vi "New Buffer.vi"(7 "byte order (host order)":T1(ring)=enum."native, host order", 8 "error in (no error)":errorcluster, 9 "buffer offset (0)":u64 format="%d bytes", 10 "buffer size":u64 format="%d bytes", 11 "Buffer type":refnum<class "Buffer.lvclass">) -> (0 "error out":errorcluster, 3 "Buffer out":refnum<class "Buffer.lvclass">)   [LabVIEW 2021, in "DSF Core.lvlib" / "Buffer.lvclass"]
doc: "Allocates a new <b>Buffer</b> of the specified <b>Buffer type</b> that is <b>size</b> bytes in length, and with a set offset at <b>buffer offset</b>.\n\n<b>buffer offset</b> is used with the Align to Base Buffer method to change the location of <b>Buffer</b> to be aligned and offset relative to a provided base Buffer."
uses:
  Buffer.lvclass
  C:/Program Files/National Instruments/LabVIEW 2021/vi.lib/NI/Memory Manager/Classes/Pointer/Pointer.lvclass
  Buffer.lvclass/Buffer.ctl
  <vilib>/NI/Memory Manager/Classes/Pointer/Pointer.lvclass/Pointer.ctl
  <vilib>/NI/Memory Manager/Classes/Pointer/Set Address.vi
  <vilib>/NI/Memory Manager/Classes/Pointer/Set Size.vi
  <vilib>/NI/Memory Manager/Classes/Pointer/Set Internal.vi
  <vilib>/NI/Memory Manager/Classes/Pointer/Pointer.lvclass
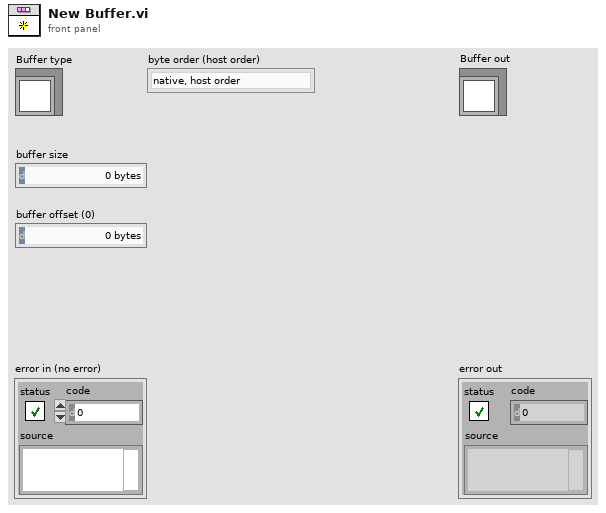
[diagram p1: front panel]
types:
  T1 = enum16{"big-endian, network order", "native, host order", "little-endian"}
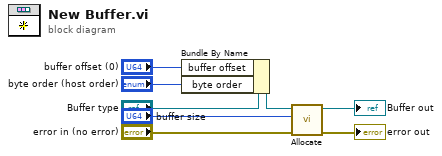
[diagram p0: block diagram]
diagram:
  n1 = Bundle By Name(cluster="Buffer type", "buffer offset"="buffer offset (0)", "byte order"="byte order (host order)") -> (w5:refnum<class "Buffer.lvclass">)
  n2 = call <vilib>:"Allocate.vi"("error in (no error)"="error in (no error)", "size"="buffer size", "Pointer type"=w5) -> ("error out"=→"error out":errorcluster, "Pointer out"=→"Buffer out":refnum<class "Buffer.lvclass">)  [unwired: 7 in]
